vi "Read Echarpe Status.vi"(8 "error in (no error)":errorcluster, 11 "Application in":refnum<class "Application.lvclass">) -> (0 "error out":errorcluster, 2 "Header Contents out":T1={"FILENAME"=["FILENAME", "example.fits", "File name at acquisition"], "OBSERVER"=["OBSERVER", "ECHARPE", "PI name"], "PROGRID"=["PROGRID", "UNDEFINED", "Program ID"], "OBJECT"=["OBJECT", "UNDEFINED", "Object name"], "NIGHTDIR"=["NIGHTDIR", "C:\\Users\\Sparc4_2\\Desktop\\Software Echarpe\\Imagens", "Night directory name "], "CHANNEL"=["CHANNEL", "RED", "Instrument channel"], "INSTRUME"=["INSTRUME", "ECHARPE", "Instrument"], "NEXPSEQ"=["NEXPSEQ", "1", "Total number of exposures in sequence"], "SEQINDEX"=["SEQINDEX", "1", "Exposure index in the sequence"], "OBSTYPE"=["OBSTYPE", "BIAS", "Image type: OBJECT, BIAS, FLAT, ARC, DARK"], "READMOD"=["READMOD", "Normal", "Read out mode: fast, normal, slow"], "SHUTTER"=["SHUTTER", "CLOSED", "Shutter Mode (OPEN, CLOSED, or AUTO) "], "OPENSHT"=["OPENSHT", "50", "Time to open the shutter (ms) "], "CLOSESHT"=["CLOSESHT", "50", "Time to close the shutter (ms)"], "GAIN"=["GAIN", "3.38", "Gain (e-/ADU)"], "GAINERR "=["GAINERR", "0.05", " Gain error (e-/ADU)"], "RDNOISE"=["RDNOISE", "6.55", "Read noise (e-)"], "RNOISERR"=["RNOISERR", "0.02", "Read noise error (e-)"], "SKYFIBER"=["SKYFIBER", "OFF", "Sky fiber: ON or OFF"], "CALFIBER"=["CALFIBER", "OFF", "Calibration Fiber: ON or OFF"], "UTDATE"=["UTDATE", "2017-10-01T20", "UT date at start of exposure"], "LOCTIME"=["LOCTIME", "2017-10-01T17", "LT date at start of exposure"], "MJD"=["MJD", "58027.500000", "Modified Julian Date at start of exposure"], "OBSLON"=["OBSLON", "-45.57972", "Observatory East Longitude"], "OBSLAT"=["OBSLAT", "-22.53444", "Observatory Latitude"], "OBSALT"=["OBSALT", "1864.0", "Observatory elevation above sea level (m)"], "EXPTIME"=["EXPTIME", "1", "Exposure time (s)"], "TELRA"=["TELRA", "00:00:00.000", "TCS right ascension: HH:MM:SS.SSS"], "TELDEC"=["TELDEC", "+00:00:00.000", "TCS declination: +-DD:MM:SS.SSS"], "RA"=["RA", "00:00:00.000", "Requested right Ascension: HH:MM:SS.SSS"], "DEC"=["DEC", "+00:00:00.000", "Requested Declination: +- DD:MM:SS.SSS"], "RA_DEG"=["RA_DEG", "128.84946", "Requested Right Ascension (deg)"], "DEC_DEG"=["DEC_DEG", "+19.648717", "Requested Declination (deg)"], "EPOCH"=["EPOCH", "2000.00", "Epoch for Target coordinates"], "HA"=["HA", "+01:13:05.98", "Hour Angle (Sexagesimal)"], "HAD"=["HAD", "1.2183292", "Hour Angle (deg)"], "AIRMASS"=["AIRMASS", "1.085", "Mean airmass for the observation"], "AMSTART"=["AMSTART", "1.060", "Airmass at start of exposure"], "AMEND"=["AMEND", "1.114", "Airmass at end of exposure"], "XOFFSET"=["XOFFSET", "0.000000", "Telescope RA offset in arcsec"], "YOFFSET"=["YOFFSET", "0.000000", "Telescope DEC offset in arcsec"], "PA"=["PA", "14.6415392418", "Current Rotator Position Angle (degree)"], "CAMFOC"=["CAMFOC", "-3.53", "Camera focus position (mm)"], "TELFOC"=["TELFOC", "-3.53", "Telescope focus position (mm)"], "TCSUT"=["TCSUT", "23:17:24.8", "TCS Universal Time"], "MOONDIST"=["MOONDIST", "60.0", "Moon angular distance to object (deg)"], "MOONALT"=["MOONALT", "15.0", "Moon elevation above horizon (deg)"], "MONNPHAS"=["MOONPHAS", "30.0", "Moon phase (deg)"], "ADC"=["ADC", "ON", "Atmospheric Dispersion Corrector: ON or OFF"], "ADCSPPED"=["ADCSPPED", "5.0", "ADC motor speed (rpm)"], "CALMIRR"=["CALMIRR", "OUT", "Calibration mirror position: IN or OUT"], "GUIDING"=["GUIDING", "ON", "Guider status: ON or OFF"], "GUIDTEXP"=["GUIDTEXP", "1.0", "Guider exposure time (s)"], "GUIDFREQ"=["GUIDFREQ", "1.0", "Guiding frequency (Hz)"], "GUIDOBJX"=["GUIDOBJX", "102.5", "Guiding object x position (pixel)"], "GUIDOBJY"=["GUIDOBJY", "300.3", "Guiding object y position (pixel)"], "AVGYCORR"=["AVGYCORR", "2.3", "Average correction in RA (arcsec)"], "AVGXCORR"=["AVGXCORR", "1.3", "Average correction in DEC (arcsec)"], "GFOCUS"=["GFOCUS", "3.0", "Guider focus position (mm)"], "THARLAMP"=["THARLAMP", "OFF", "Thorium-Argon lamp state: ON or OFF"], "HALLAMP"=["HALLAMP", "OFF", "Halogen lamp state: ON or OFF"], "AGITATOR"=["AGITATOR", "ON", "Fiber agitator: ON or OFF"], "THARMIRR"=["THARMIRR", "SPECTROGRAPH", "Th-Ar mirror position: SPECTROGRAPH or TELESCOPE"], "DSTATUS"=["DSTATUS", "OPEN", "Dome Status: OPEN or CLOSED"], "DTEMP"=["DTEMP", "10.0", "Dome temperature (deg C)"], "DHUM"=["DHUM", "82.0", "Dome humidity (per cent)"], "DLAMP"=["DLAMP", "OFF", "Dome lamp: ON or OFF"], "DFLAT"=["DFLAT", "OFF", "Dome flat lamp: ON or OFF"], "TEMPEXT"=["TEMPEXT", "10.0", "External temperature (deg C)"], "PRESSURE"=["PRESSURE", "742.00", "Pressure (mbar)"], "HUMIDITY"=["HUMIDITY", "92.00", "Humidity (per cent)"], "WINDDIR"=["WINDDIR", "15.0", "Wind direction: North-eastward (deg)"], "WSPEED"=["WSPEED", "30.2", "Wind Speed (km/h)"], "TCSST"=["TCSST", "23:12:32.5", "TCS Sideral Time"], "DPOS"=["DPOS", "0.00000", "Dome position (deg)"]}, 3 "Application out":refnum<class "Application.lvclass">)   [LabVIEW 2018, in "Application.lvclass"]
doc: "Este VI realiza a leitura do status de todos os objetos referentes ao uso do instrumento. O cluster Header Contents e passado por cada objeto e, ao final, obtém-se o conjunto de informações necessárias para a escrita do header da imagem."
uses:
  Application.lvclass
  Application.lvclass/Application.ctl
  User/User.lvclass
  TCS/TCS.lvclass
  Guider/Guider.lvclass
  Calibration Unit/Calibration Unit.lvclass
  Weather Station/Weather Station.lvclass
  Fore Optics/Fore Optics.lvclass
  Dome/Dome.lvclass
  CCDCamera/CCDCamera.lvclass
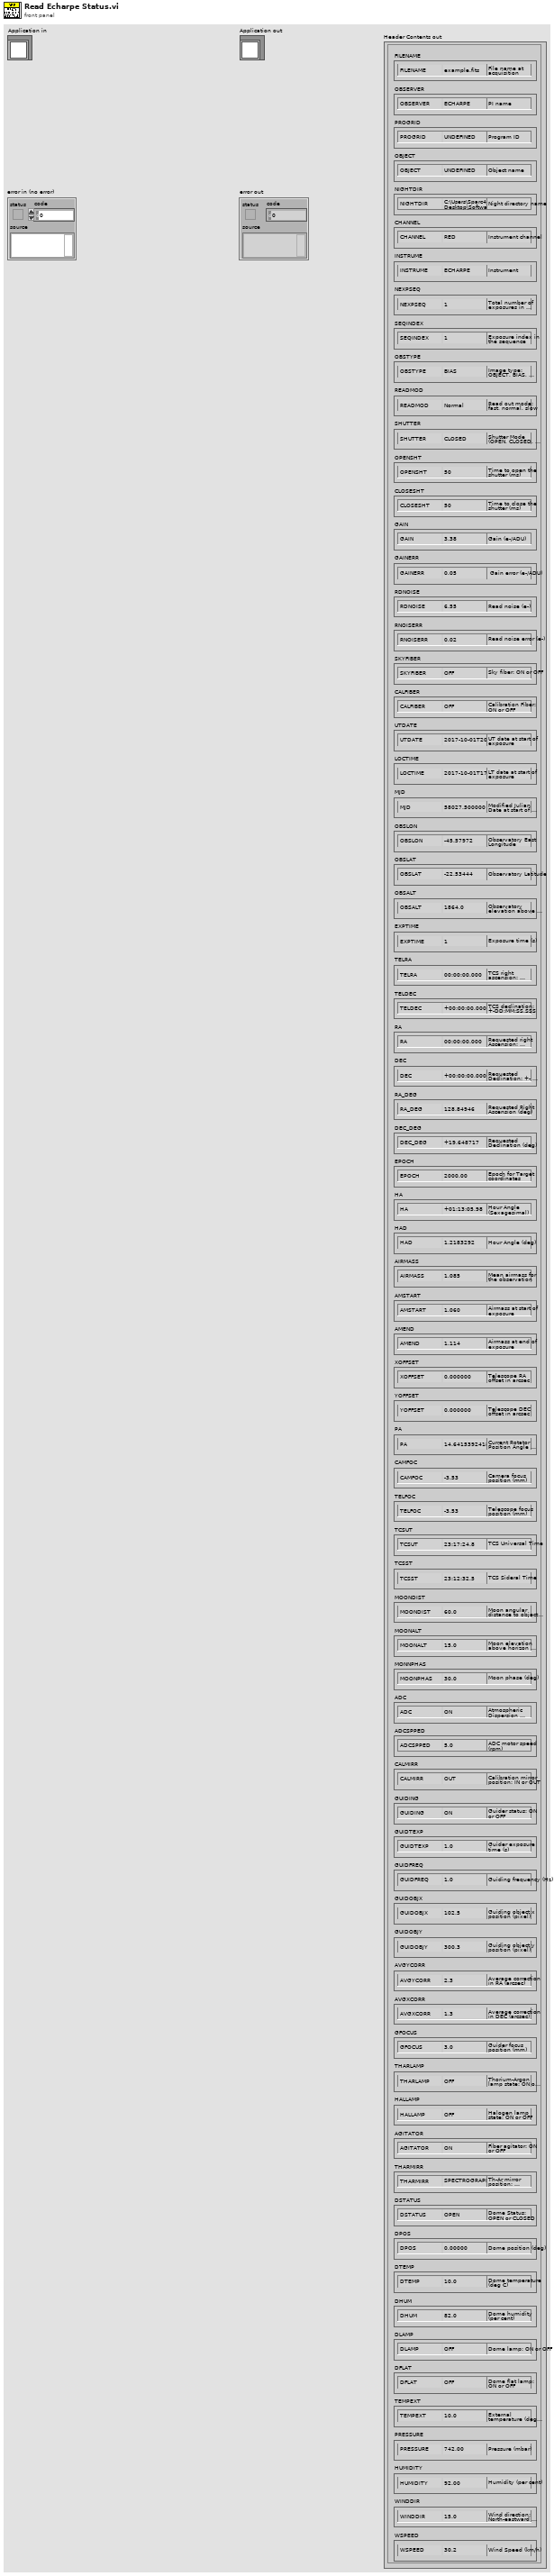
[diagram p1: front panel]
types:
  T1 = cluster{"FILENAME":string[], "OBSERVER":string[], "PROGRID":string[], "OBJECT":string[], "NIGHTDIR":string[], "CHANNEL":string[], "INSTRUME":string[], "NEXPSEQ":string[], "SEQINDEX":string[], "OBSTYPE":string[], "READMOD":string[], "SHUTTER":string[], "OPENSHT":string[], "CLOSESHT":string[], "GAIN":string[], "GAINERR ":string[], "RDNOISE":string[], "RNOISERR":string[], "SKYFIBER":string[], "CALFIBER":string[], "UTDATE":string[], "LOCTIME":string[], "MJD":string[], "OBSLON":string[], "OBSLAT":string[], "OBSALT":string[], "EXPTIME":string[], "TELRA":string[], "TELDEC":string[], "RA":string[], "DEC":string[], "RA_DEG":string[], "DEC_DEG":string[], "EPOCH":string[], "HA":string[], "HAD":string[], "AIRMASS":string[], "AMSTART":string[], "AMEND":string[], "XOFFSET":string[], "YOFFSET":string[], "PA":string[], "CAMFOC":string[], "TELFOC":string[], "TCSUT":string[], "MOONDIST":string[], "MOONALT":string[], "MONNPHAS":string[], "ADC":string[], "ADCSPPED":string[], "CALMIRR":string[], "GUIDING":string[], "GUIDTEXP":string[], "GUIDFREQ":string[], "GUIDOBJX":string[], "GUIDOBJY":string[], "AVGYCORR":string[], "AVGXCORR":string[], "GFOCUS":string[], "THARLAMP":string[], "HALLAMP":string[], "AGITATOR":string[], "THARMIRR":string[], "DSTATUS":string[], "DTEMP":string[], "DHUM":string[], "DLAMP":string[], "DFLAT":string[], "TEMPEXT":string[], "PRESSURE":string[], "HUMIDITY":string[], "WINDDIR":string[], "WSPEED":string[], "TCSST":string[], "DPOS":string[]}
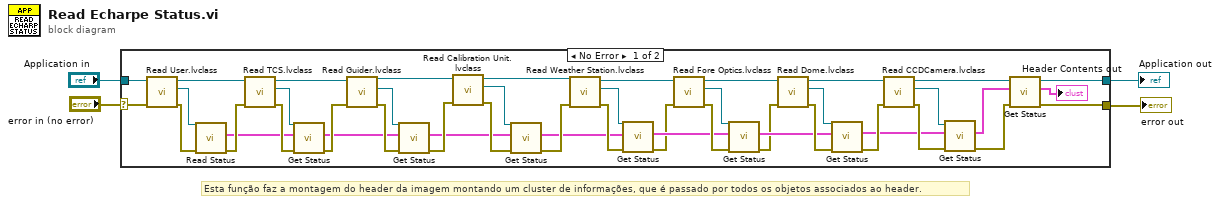
[diagram p0: block diagram]
diagram:
  # "Esta função faz a montagem do header da imagem montando um cluster de informações, que é passado por todos os objetos associados ao header."
  n1 = case shown="No Error" "error in (no error)" {
    selector: "error in (no error)" -> [w49 w51]
    tunnel: [w41 w51] -> w3
    tunnel: [w43 w50] -> w1
    tunnel: "Application in" -> [w44 w50]
    frame No Error {
      n2 = call "Read User.lvclass.vi"("error in (no error)"=w49, "Application in"=w44) -> ("error out"=w48:errorcluster, "User.lvclass"=w39:refnum<class "User.lvclass">, "Application out"=w42:refnum<class "Application.lvclass">)  [unwired: 7 in]
      n3 = call "Read Status.vi"("error in (no error)"=w48, "User in"=w39) -> ("error out"=w47:errorcluster, "Header Contents out"=w38:T1)  [unwired: 7 in, 1 out]
      n4 = call "Read TCS.lvclass.vi"("error in (no error)"=w47, "Application in"=w42) -> ("error out"=w46:errorcluster, "TCS.lvclass"=w45:refnum<class "TCS.lvclass">, "Application out"=w36:refnum<class "Application.lvclass">)  [unwired: 7 in]
      n5 = call "Get Status.vi"("error in (no error)"=w46, "Header Contents in"=w38, "TCS in"=w45) -> ("error out"=w37:errorcluster, "Header Contents out"=w34:T1)  [unwired: 6 in, 1 out]
      n6 = call "Read Guider.lvclass.vi"("error in (no error)"=w37, "Application in"=w36) -> ("error out"=w35:errorcluster, "Guider.lvclass"=w33:refnum<class "Guider.lvclass">, "Application out"=w31:refnum<class "Application.lvclass">)  [unwired: 7 in]
      n7 = call "Get Status.vi"("error in (no error)"=w35, "Header Contents in"=w34, "Guider in"=w33) -> ("error out"=w32:errorcluster, "Header Contents out"=w29:T1)  [unwired: 6 in, 1 out]
      n8 = call "Read Calibration Unit.lvclass.vi"("error in (no error)"=w32, "Application in"=w31) -> ("error out"=w30:errorcluster, "Calibration Unit.lvclass"=w28:refnum<class "Calibration Unit.lvclass">, "Application out"=w13:refnum<class "Application.lvclass">)  [unwired: 7 in]
      n9 = call "Get Status.vi"("error in (no error)"=w30, "Header Contents in"=w29, "Calibration Unit in"=w28) -> ("error out"=w15:errorcluster, "Header Contents out"=w14:T1)  [unwired: 6 in, 1 out]
      n10 = call "Read Weather Station.lvclass.vi"("error in (no error)"=w15, "Application in"=w13) -> ("error out"=w19:errorcluster, "Weather Station.lvclass"=w18:refnum<class "Weather Station.lvclass">, "Application out"=w16:refnum<class "Application.lvclass">)  [unwired: 7 in]
      n11 = call "Get Status.vi"("error in (no error)"=w19, "Header Contents in"=w14, "Weather Station in"=w18) -> ("error out"=w20:errorcluster, "Header Contents out"=w21:T1)  [unwired: 6 in, 1 out]
      n12 = call "Read Fore Optics.lvclass.vi"("error in (no error)"=w20, "Application in"=w16) -> ("error out"=w22:errorcluster, "Fore Optics.lvclass"=w24:refnum<class "Fore Optics.lvclass">, "Application out"=w17:refnum<class "Application.lvclass">)  [unwired: 7 in]
      n13 = call "Get Status.vi"("error in (no error)"=w22, "Header Contents in"=w21, "Fore Optics in"=w24) -> ("error out"=w23:errorcluster, "Header Contents out"=w25:T1)  [unwired: 6 in, 1 out]
      n14 = call "Read Dome.lvclass.vi"("error in (no error)"=w23, "Application in"=w17) -> ("error out"=w27:errorcluster, "Dome.lvclass"=w26:refnum<class "Dome.lvclass">, "Application out"=w11:refnum<class "Application.lvclass">)  [unwired: 7 in]
      n15 = call "Get Status.vi"("error in (no error)"=w27, "Header Contents in"=w25, "Dome in"=w26) -> ("error out"=w12:errorcluster, "Header Contents out"=w8:T1)  [unwired: 6 in, 1 out]
      n16 = call "Read CCDCamera.lvclass.vi"("error in (no error)"=w12, "Application in"=w11) -> ("error out"=w10:errorcluster, "CCDCamera.lvclass"=w9:refnum<class "CCDCamera.lvclass">, "Application out"=w6:refnum<class "Application.lvclass">)  [unwired: 7 in]
      n17 = call "Get Status.vi"("error in (no error)"=w10, "Header Contents in"=w8, "CCDCamera in"=w9) -> ("error out"=w5:errorcluster, "Header Contents out"=w7:T1)  [unwired: 6 in, 1 out]
      n18 = call "Get Status.vi"("error in (no error)"=w5, "Header Contents in"=w7, "Application in"=w6) -> ("error out"=w41:errorcluster, "Header Contents out"=→"Header Contents out":T1, "Application out"=w43:refnum<class "Application.lvclass">)  [unwired: 6 in]
    }
    frame Error {
    }
  }
  "error out" <- w3
  "Application out" <- w1
